vi "elevador.vi"() -> ()   [LabVIEW 2020]
panel:
  out "Boolean 8":bool
  out "Boolean 10":bool
  out "Boolean 9":bool
  out "Boolean 11":bool
  out "Boolean 7":bool
  out "Boolean 6":bool
  out "Boolean 3":bool
  in  "puerta elevador":bool
  out "elevador":bool
  in  "piso":u8 max=3 step=1
  in  "stop":bool
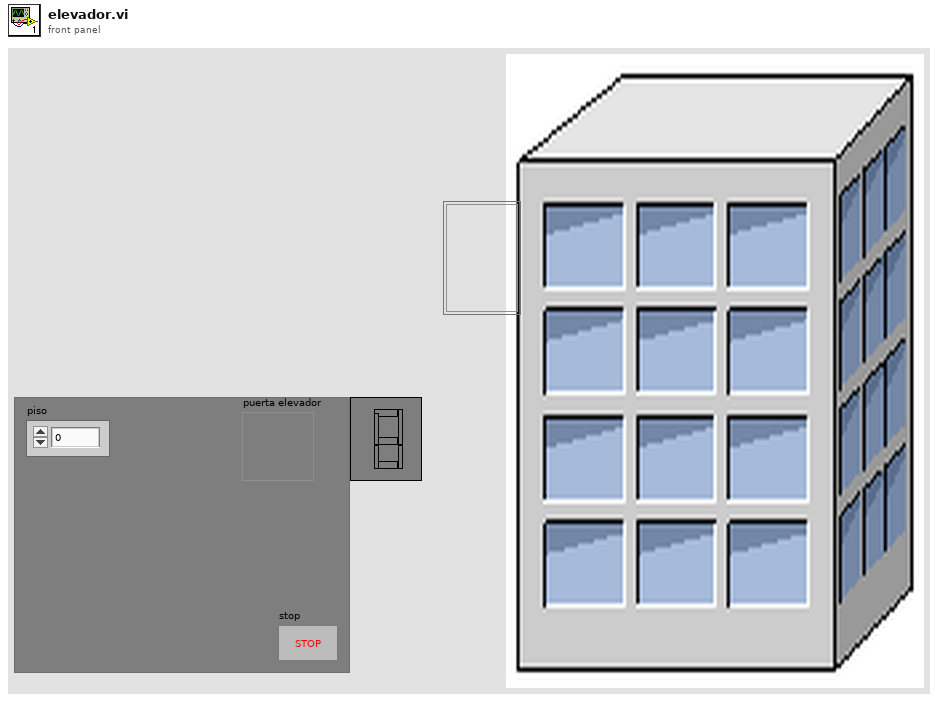
[diagram p1: front panel]
types:
  T1 = enum16{"Estatico", "Desicion", "subir", "bajar", "puerta"}
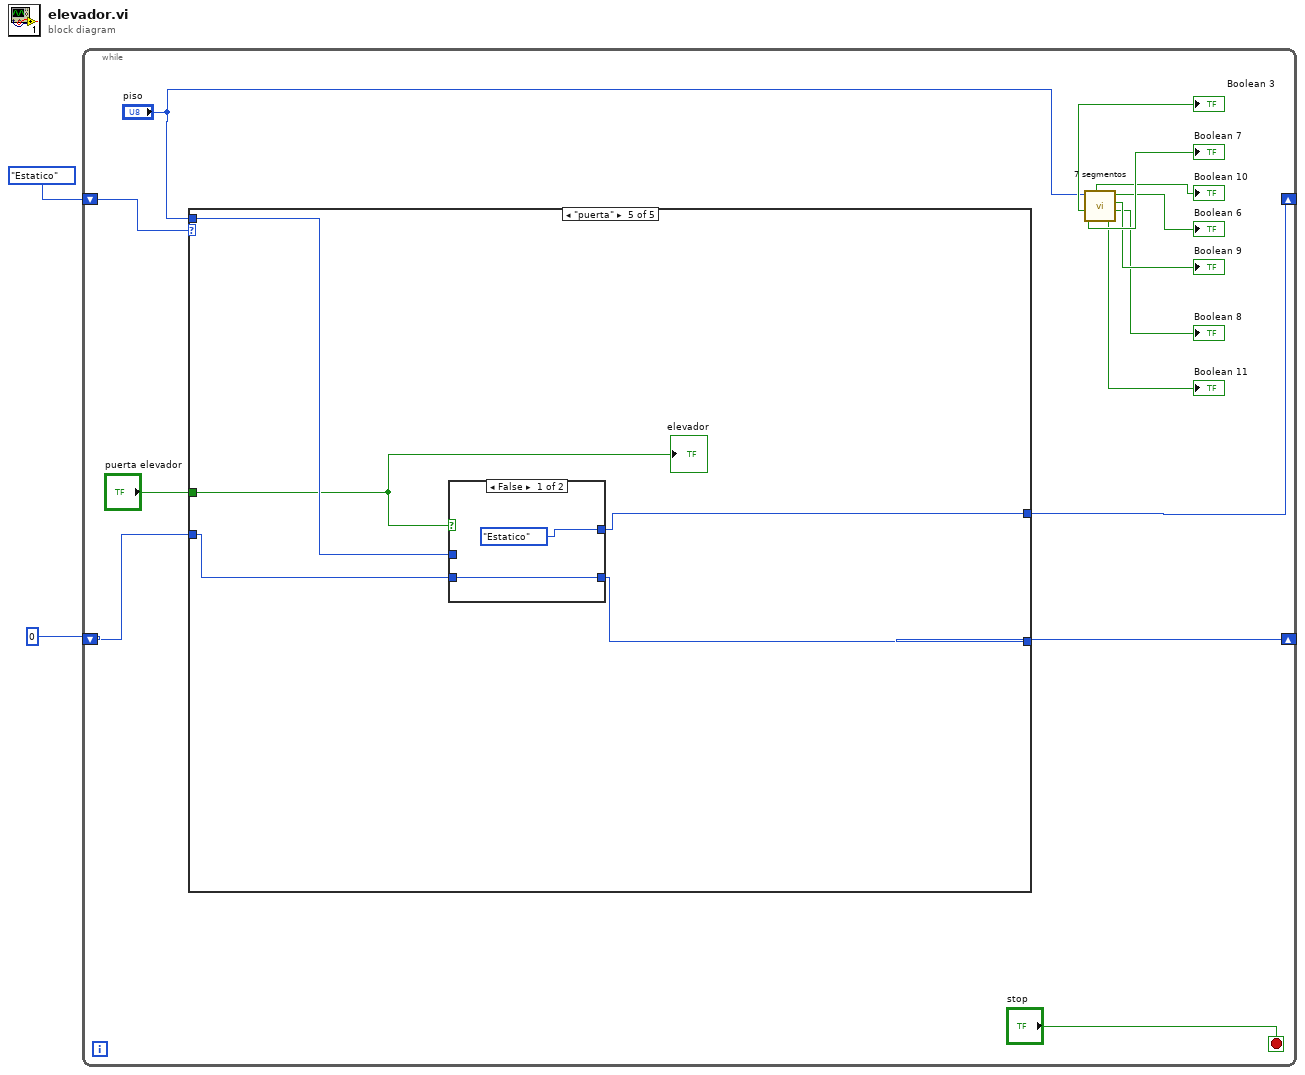
[diagram p0: block diagram]
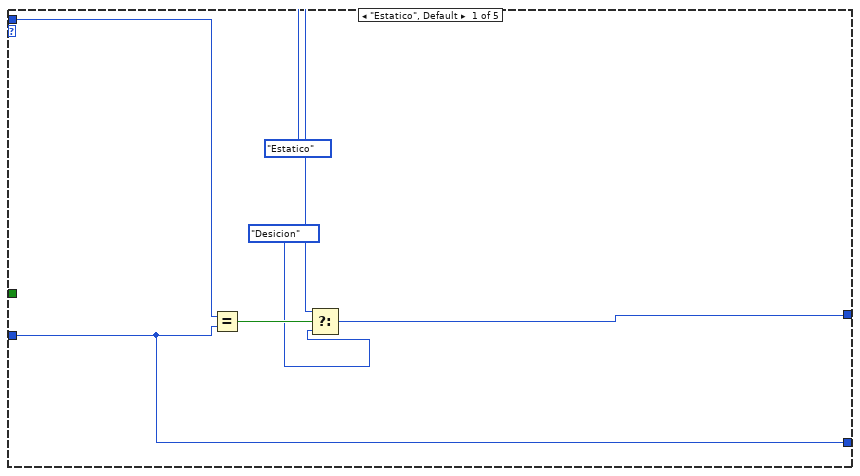
[diagram p2: hidden frame]
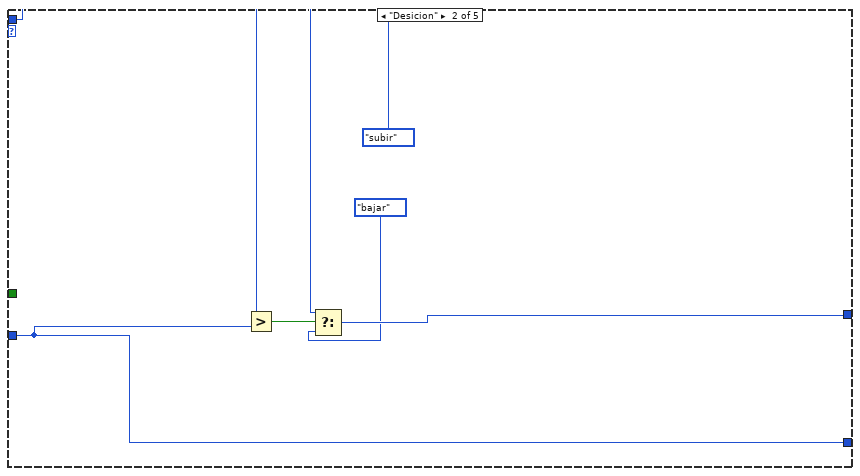
[diagram p3: hidden frame]
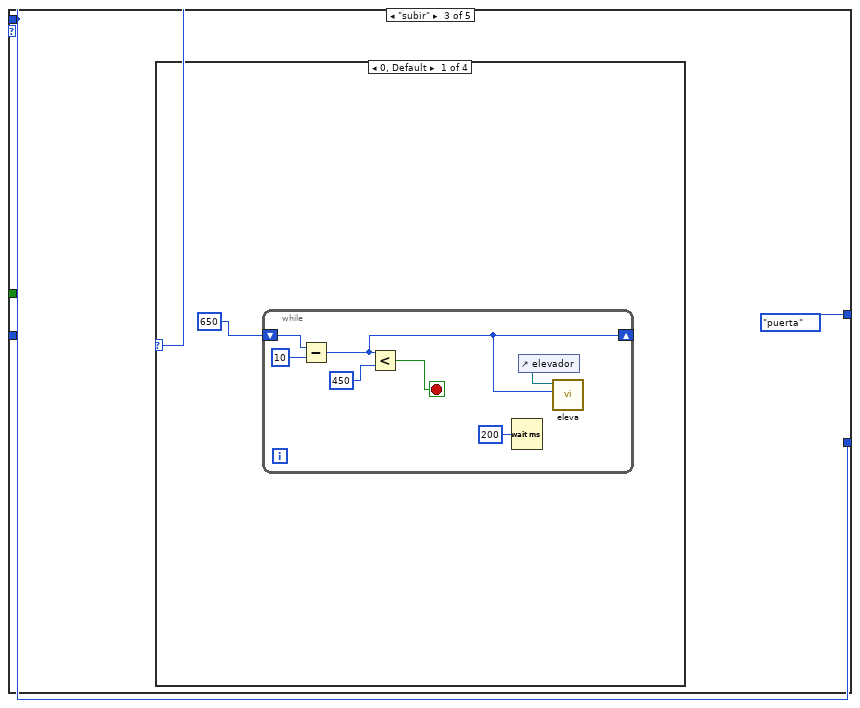
[diagram p4: hidden frame]
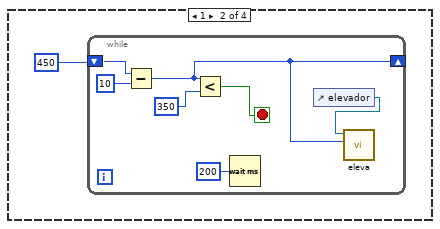
[diagram p5: hidden frame]
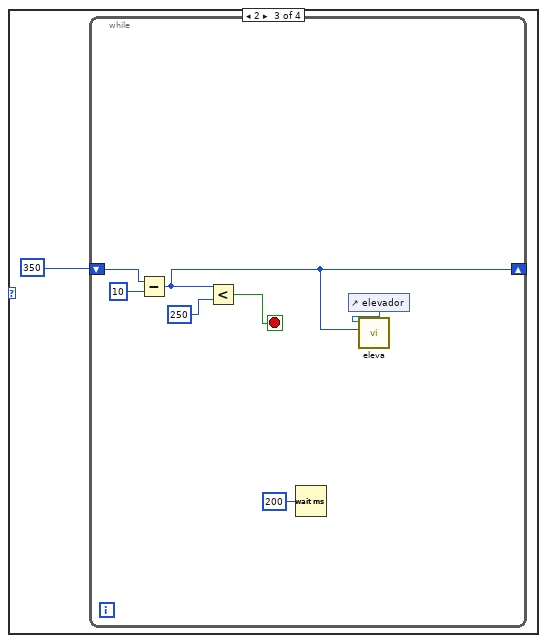
[diagram p6: hidden frame]
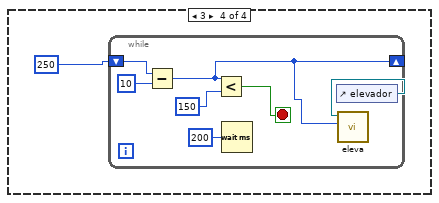
[diagram p7: hidden frame]
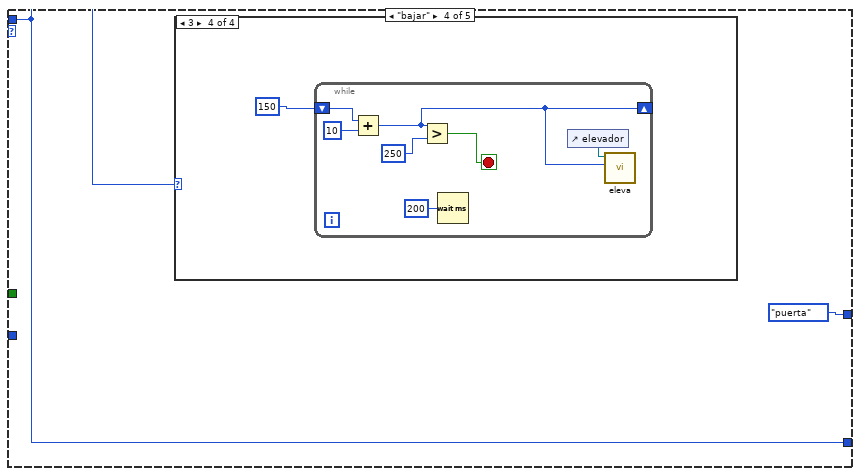
[diagram p8: hidden frame]
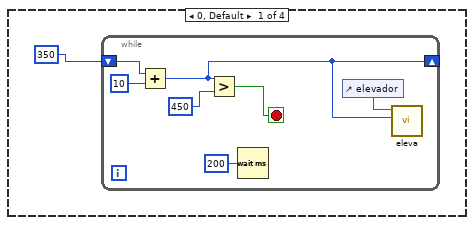
[diagram p9: hidden frame]
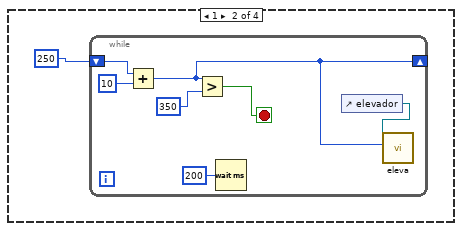
[diagram p10: hidden frame]
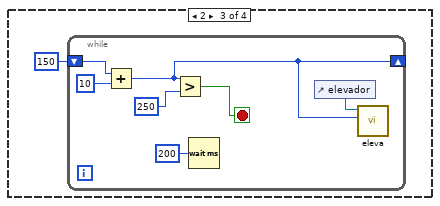
[diagram p11: hidden frame]
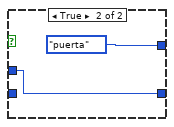
[diagram p12: hidden frame]
diagram:
  n1 = while {
    shift-right: [w14] -> _
    shift-left: T1."Estatico" -> [w16]
    shift-right: [w12] -> _
    shift-left: 0 -> [w13]
    stop <- "stop" stop-if-true
    n2 = case shown="\"puerta\"" w16 {
      tunnel: "piso" -> [w17 w23 w29 w63 w100]
      tunnel: w13 -> [w19 w24 _ _ w99]
      tunnel: [w18 w27 T1."puerta" T1."puerta" w101] -> w14
      tunnel: [w19 w24 w29 w63 w98] -> w12
      tunnel: "puerta elevador" -> [_ _ _ _ w97]
      frame "Estatico", Default {
        n3 = Equal?(x=w17, y=w19) -> (x = y?=w22:bool)
        n4 = Select(t=T1."Estatico", s=w22, f=T1."Desicion") -> (s? t:f=w18:T1)
      }
      frame "Desicion" {
        n5 = Greater?(x=w23, y=w24) -> (0:w28:bool)
        n6 = Select(t=T1."subir", s=w28, f=T1."bajar") -> (s? t:f=w27:T1)
      }
      frame "subir" {
        n7 = case shown="0, Default" w29 {
          frame 0, Default {
            n8 = while {
              shift-right: [w33] -> _
              shift-left: 650 -> [w38]
              stop <- w35 stop-if-true
              n9 = Subtract(x=w38, y=10) -> (x-y=w33:i32)
              n10 = Less?(x=w33, y=450) -> (x < y?=w35:bool)
              n11 = Wait (ms)(milliseconds to wait=u32 200) -> ()  [unwired: 1 out]
              n12 = control-ref of="elevador"() -> (w34:refnum<vi>)
              n13 = call "eleva.vi"("Position:Top"=w33, "Boolean in"=w34) -> ()  [unwired: 10 in]
            }
          }
          frame 1 {
            n14 = while {
              shift-right: [w41] -> _
              shift-left: 450 -> [w46]
              stop <- w43 stop-if-true
              n15 = Subtract(x=w46, y=10) -> (x-y=w41:i32)
              n16 = Less?(x=w41, y=350) -> (x < y?=w43:bool)
              n17 = Wait (ms)(milliseconds to wait=u32 200) -> ()  [unwired: 1 out]
              n18 = control-ref of="elevador"() -> (w42:refnum<vi>)
              n19 = call "eleva.vi"("Position:Top"=w41, "Boolean in"=w42) -> ()  [unwired: 10 in]
            }
          }
          frame 2 {
            n20 = while {
              shift-right: [w49] -> _
              shift-left: 350 -> [w54]
              stop <- w51 stop-if-true
              n21 = Subtract(x=w54, y=10) -> (x-y=w49:i32)
              n22 = Less?(x=w49, y=250) -> (x < y?=w51:bool)
              n23 = Wait (ms)(milliseconds to wait=u32 200) -> ()  [unwired: 1 out]
              n24 = control-ref of="elevador"() -> (w50:refnum<vi>)
              n25 = call "eleva.vi"("Position:Top"=w49, "Boolean in"=w50) -> ()  [unwired: 10 in]
            }
          }
          frame 3 {
            n26 = while {
              shift-right: [w57] -> _
              shift-left: 250 -> [w62]
              stop <- w59 stop-if-true
              n27 = Subtract(x=w62, y=10) -> (x-y=w57:i32)
              n28 = Less?(x=w57, y=150) -> (x < y?=w59:bool)
              n29 = Wait (ms)(milliseconds to wait=u32 200) -> ()  [unwired: 1 out]
              n30 = control-ref of="elevador"() -> (w58:refnum<vi>)
              n31 = call "eleva.vi"("Position:Top"=w57, "Boolean in"=w58) -> ()  [unwired: 10 in]
            }
          }
        }
      }
      frame "bajar" {
        n32 = case shown="3" w63 {
          frame 0, Default {
            n33 = while {
              shift-right: [w68] -> _
              shift-left: 350 -> [w72]
              stop <- w69 stop-if-true
              n34 = Add(x=w72, y=10) -> (x+y=w68:i32)
              n35 = Greater?(x=w68, y=450) -> (0:w69:bool)
              n36 = Wait (ms)(milliseconds to wait=u32 200) -> ()  [unwired: 1 out]
              n37 = control-ref of="elevador"() -> (w67:refnum<vi>)
              n38 = call "eleva.vi"("Position:Top"=w68, "Boolean in"=w67) -> ()  [unwired: 10 in]
            }
          }
          frame 1 {
            n39 = while {
              shift-right: [w76] -> _
              shift-left: 250 -> [w80]
              stop <- w77 stop-if-true
              n40 = Add(x=w80, y=10) -> (x+y=w76:i32)
              n41 = Greater?(x=w76, y=350) -> (0:w77:bool)
              n42 = Wait (ms)(milliseconds to wait=u32 200) -> ()  [unwired: 1 out]
              n43 = control-ref of="elevador"() -> (w75:refnum<vi>)
              n44 = call "eleva.vi"("Position:Top"=w76, "Boolean in"=w75) -> ()  [unwired: 10 in]
            }
          }
          frame 2 {
            n45 = while {
              shift-right: [w84] -> _
              shift-left: 150 -> [w88]
              stop <- w85 stop-if-true
              n46 = Add(x=w88, y=10) -> (x+y=w84:i32)
              n47 = Greater?(x=w84, y=250) -> (0:w85:bool)
              n48 = Wait (ms)(milliseconds to wait=u32 200) -> ()  [unwired: 1 out]
              n49 = control-ref of="elevador"() -> (w83:refnum<vi>)
              n50 = call "eleva.vi"("Position:Top"=w84, "Boolean in"=w83) -> ()  [unwired: 10 in]
            }
          }
          frame 3 {
            n51 = while {
              shift-right: [w92] -> _
              shift-left: 150 -> [w96]
              stop <- w93 stop-if-true
              n52 = Add(x=w96, y=10) -> (x+y=w92:i32)
              n53 = Greater?(x=w92, y=250) -> (0:w93:bool)
              n54 = Wait (ms)(milliseconds to wait=u32 200) -> ()  [unwired: 1 out]
              n55 = control-ref of="elevador"() -> (w91:refnum<vi>)
              n56 = call "eleva.vi"("Position:Top"=w92, "Boolean in"=w91) -> ()  [unwired: 10 in]
            }
          }
        }
      }
      frame "puerta" {
        n57 = case shown="False" w97 {
          tunnel: [T1."Estatico" T1."puerta"] -> w101
          tunnel: w100 -> [_ w104]
          tunnel: w99 -> [w102 _]
          tunnel: [w102 w104] -> w98
          frame False {
          }
          frame True {
          }
        }
        "elevador" <- w97
      }
    }
    n58 = call "7 segmentos.vi"("Numeric"="piso") -> ("[6]"=→"Boolean 11":bool, "[5]"=→"Boolean 8":bool, "[4]"=→"Boolean 9":bool, "[3]"=→"Boolean 6":bool, "[2]"=→"Boolean 10":bool, "[1]"=→"Boolean 7":bool, "[0]"=→"Boolean 3":bool)  [unwired: 1 in]
  }
